vi "Broker.vi"() -> ()   [LabVIEW 2019]
uses:
  <vilib>/LabVIEW Open Source Project/MQTT TCP Connection/MQTT_TCP/Connection/TCPConnection.lvclass
  <vilib>/G Open Source Project for LabVIEW/MQTT Broker/Server class/Server.lvclass
  <vilib>/LabVIEW Open Source Project/MQTT Connection/MQTT_Base/Base Class/MQTT_Base.lvclass
  C:/Program Files (x86)/National Instruments/LabVIEW 2019/vi.lib/LabVIEW Open Source Project/MQTT Connection/MQTT_Connection/Connection/Connection.lvclass
  C:/Program Files (x86)/National Instruments/LabVIEW 2019/vi.lib/LabVIEW Open Source Project/MQTT Connection/MQTT_Base/Base Class/MQTT_Base.lvclass
panel:
  in  "error in (no error)":errorcluster
  out "Connected Clients":u64
  in  "stop":bool
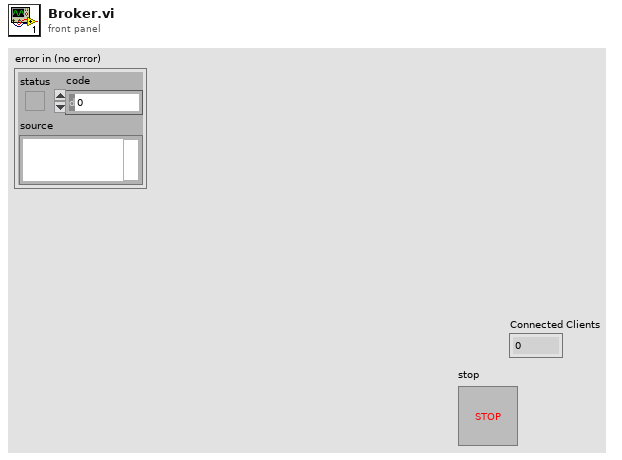
[diagram p1: front panel]
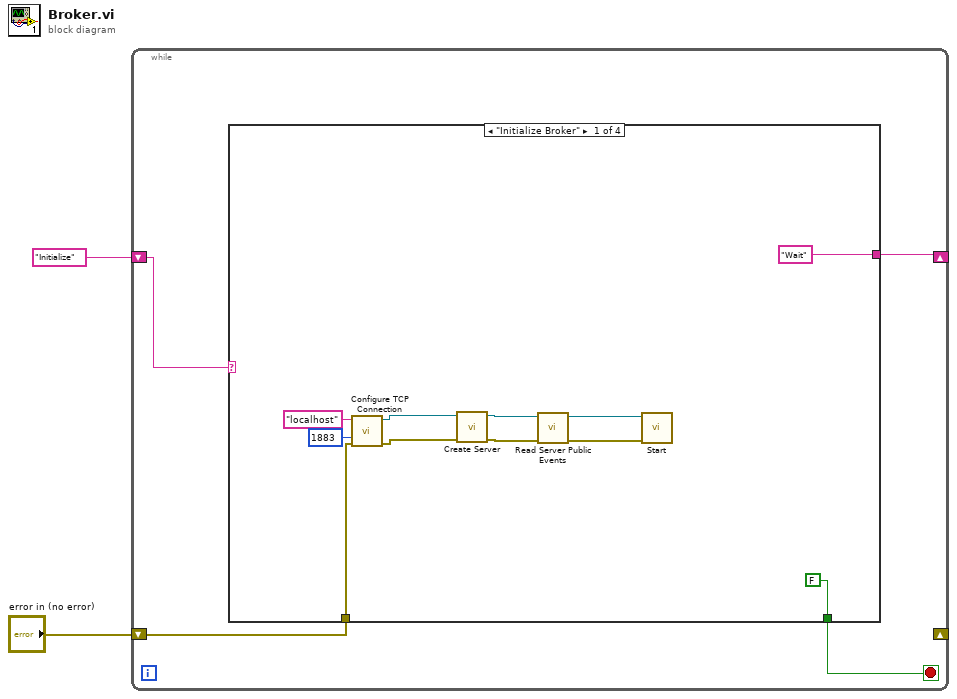
[diagram p0: block diagram]
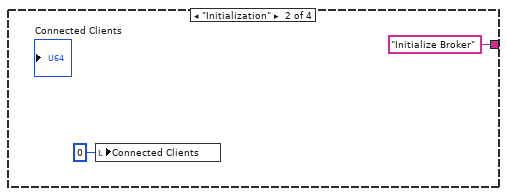
[diagram p2: hidden frame]
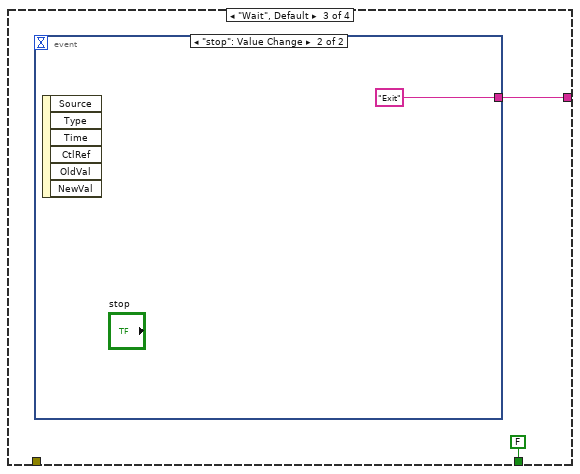
[diagram p3: hidden frame]
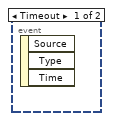
[diagram p4: hidden frame]
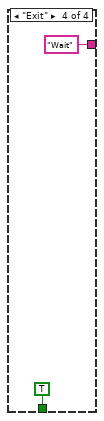
[diagram p5: hidden frame]
diagram:
  n1 = while {
    shift-right: [w5] -> _
    shift-left: "Initialize" -> [w6]
    shift-right: _ -> [_]
    shift-left: "error in (no error)" -> [w3]
    stop <- w4 stop-if-true
    n2 = case shown="\"Initialize Broker\"" w6 {
      tunnel: ["Wait" "Initialize Broker" w21 "Wait"] -> w5
      tunnel: [FALSE _ FALSE TRUE] -> w4
      tunnel: w3 -> [w13 _ _ _]
      frame "Initialize Broker" {
        n3 = call <vilib>:"Configure TCP Connection.vi"("error in (no error)"=w13, "remote port (80)"=u16 1883, "address (localhost)"="localhost") -> ("error out"=w11:errorcluster, "TCPConnection"=w12:refnum<class "TCPConnection.lvclass">)  [unwired: 7 in]
        n4 = call <vilib>:"Create Server.vi"("error in (no error)"=w11, "Connection Configuration"=w12) -> ("error out"=w9:errorcluster, "Server"=w10:refnum<class "Server.lvclass">)  [unwired: 8 in]
        n5 = call <vilib>:"Read Server Public Events.vi"("error in (no error)"=w9, "Server in"=w10) -> ("error out"=w7:errorcluster, "Server out"=w8:refnum<class "Server.lvclass">)  [unwired: 7 in, 1 out]
        n6 = call <vilib>:"Start.vi"("error in (no error)"=w7, "MQTT_Base in"=w8) -> ()  [unwired: 7 in, 3 out]
      }
      frame "Initialization" {
        n7 = local write "Connected Clients"(u64 0 ("Connected Clients")) -> ()
      }
      frame "Wait", Default {
        n8 = event shown="[1] \"stop\": Value Change" {
          selector: _ -> [_ _]
          dyn-events: _ -> [_ _]
          timeout: _ -> [_ _]
          tunnel: [_ "Exit"] -> w21
          event Timeout {
            n9 = event-data() -> ()  [unwired: 1 in, 3 out]
          }
          event "stop": Value Change {
            n10 = event-data() -> ()  [unwired: 1 in, 6 out]
          }
        }
      }
      frame "Exit" {
      }
    }
  }
